vi "Pre Launch Init.vi"(11 "CS++DeviceGUIActor in":refnum<class "CS++DeviceGUIActor.lvclass">) -> (0 "error out":errorcluster, 3 "CS++DeviceGUIActor out":refnum<class "CS++DeviceGUIActor.lvclass">)   [LabVIEW 2013, in "CS++DeviceGUIActor.lvlib" / "CS++DeviceGUIActor.lvclass"]
doc: "(<B>Filename</B>: Actor Framework.lvlib:Actor.lvclass:Pre Launch Init.vi)\n\nDefines behavior that occurs after the Launch Actor method is invoked but before the actor's Actor Core method begins running.\n\nThe Pre Launch Init method is guaranteed to finish before the Launch Actor method returns to its caller and before the actor itself receives any messages. Any references that the Pre Launch Init method obtains are guaranteed to have the same lifetime as the actor itself. Any errors that the Pre Launch Init method returns will abort the launch.\n\nBy default, this method does nothing. A descendant class may override it to define behavior."
uses:
  CS++DeviceGUIActor.lvclass
  CS++GUIActor/CS++GUIActor.lvclass
  CS++BaseActor/CS++BaseActor.lvclass/CS++BaseActor.ctl
  Classes/CS++BaseClasses/Factory/CS++Factory.lvclass
  Classes/CS++ProcessVariables/PVConnection/PVConnection.lvclass
  Classes/CS++ProcessVariables/ProcessVariable/PV.lvclass/PV.ctl
  CS++DeviceGUIActor.lvclass/CS++DeviceGUIActor.ctl
  Classes/CS++ProcessVariables/ProcessVariable/Read Data.vi
  CS++BaseActor/Read CS++Factory.vi
  CS++GUIActor/Read Actor Name.vi
  Classes/CS++ProcessVariables/CS++ProcessVariables.lvlib
  Classes/CS++ProcessVariables/ProcessVariable/PV.lvclass
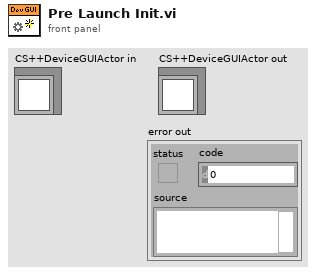
[diagram p1: front panel]
types:
  T1 = cluster{"Write Access":enum8{"Allowed", "Required", "None"}, "Read Access":enum8{"Allowed", "Required", "None"}}
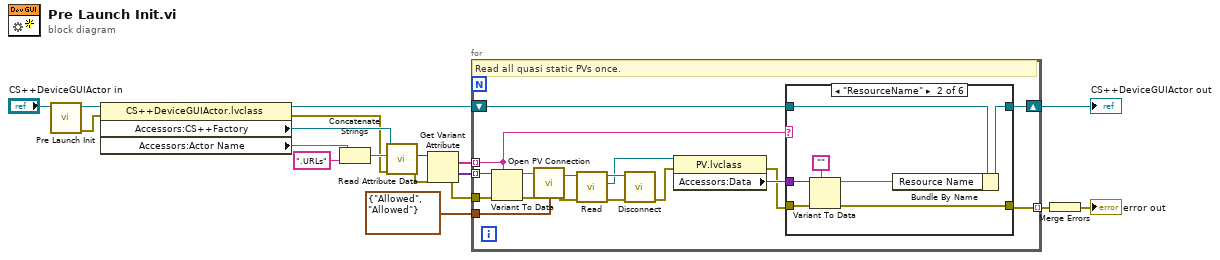
[diagram p0: block diagram]
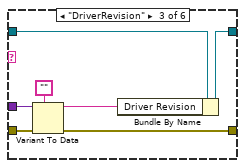
[diagram p3: hidden frame]
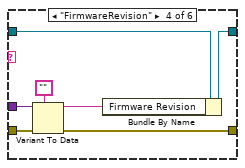
[diagram p4: hidden frame]
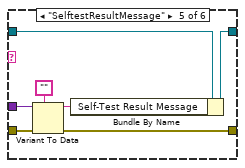
[diagram p5: hidden frame]
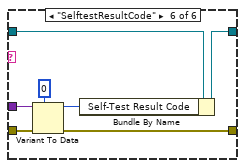
[diagram p6: hidden frame]
diagram:
  n1 = call-parent "Pre Launch Init.vi"("CS++BaseActor in"="CS++DeviceGUIActor in") -> ("error out"=w4:errorcluster, "CS++BaseActor out"=w5:refnum<class "CS++DeviceGUIActor.lvclass">)  [unwired: 9 in]
  n2 = property class="CS++DeviceGUIActor.lvclass"(reference=w5, error in=w4) -> (reference out=w7:refnum<class "CS++DeviceGUIActor.lvclass">, error out=w14:errorcluster, "Accessors:CS++Factory"=w15:refnum<class "CS++Factory.lvclass">, "Accessors:Actor Name"=w13:string)
  n3 = Concatenate Strings(w13, ".URLs" ("string")) -> (w16:string)
  n4 = call-dynamic "Read Attribute Data.vi"("error in (no error)"=w14, "Object Name"=w16, "CS++Factory in"=w15) -> ("error out"=w11:errorcluster, "Attribute Data"=w12:variant)  [unwired: 6 in, 1 out]
  n5 = Get Variant Attribute(Variant=w12, error in=w11) -> (names=w10:string[], values=w9:variant[], error out=w8:errorcluster)  [unwired: 2 in, 1 out]
  n6 = for {
    tunnel: w10 -> [w25] mode=indexing
    tunnel: w9 -> [w35] mode=indexing
    tunnel: w8 -> [w34]
    shift-right: [w32] -> w3
    shift-left: w7 -> [w33]
    tunnel: [w24] -> w6 mode=indexing
    tunnel: T1 {"Write Access"=enum."Allowed", "Read Access"=enum."Allowed"} ("Access (Read Required)") -> [w19]
    # "Read all quasi static PVs once."
    n7 = Variant To Data(error in=w34, type=w25, Variant=w35) -> (data=w23:string, error out=w22:errorcluster)
    n8 = call "Open PV Connection.vi"("PV URL"=w23, "Access (R/W allowed)"=w19, "Error In"=w22) -> ("PVConnection"=w21:refnum<class "PVConnection.lvclass">, "Error Out"=w20:errorcluster)
    n9 = call-dynamic "Read.vi"("error in (no error)"=w20, "PVConnection in"=w21) -> ("error out"=w30:errorcluster, "PV"=w29:refnum<class "PV.lvclass">, "PVConnection out"=w31:refnum<class "PVConnection.lvclass">)  [unwired: 6 in, 1 out]
    n10 = call-dynamic "Disconnect.vi"("error in (no error)"=w30, "PVConnection in"=w31) -> ("error out"=w28:errorcluster)  [unwired: 8 in, 1 out]
    n11 = property class="PV.lvclass"(reference=w29, error in=w28) -> (error out=w26:errorcluster, "Accessors:Data"=w27:variant)  [unwired: 1 out]
    n12 = case shown="\"ResourceName\"" w25 {
      tunnel: w33 -> [w37 w44 w51 w58 w65 w72]
      tunnel: [w37 w43 w50 w57 w64 w71] -> w32
      tunnel: w27 -> [_ w42 w49 w56 w63 w70]
      tunnel: w26 -> [w36 w40 w47 w54 w61 w68]
      tunnel: [w36 w38 w45 w52 w59 w66] -> w24
      frame Default {
      }
      frame "ResourceName" {
        n13 = Variant To Data(error in=w40, type="", Variant=w42) -> (data=w39:string, error out=w38:errorcluster)
        n14 = Bundle By Name(cluster=w44, "Resource Name"=w39) -> (w43:refnum<class "CS++DeviceGUIActor.lvclass">)
      }
      frame "DriverRevision" {
        n15 = Variant To Data(error in=w47, type="", Variant=w49) -> (data=w46:string, error out=w45:errorcluster)
        n16 = Bundle By Name(cluster=w51, "Driver Revision"=w46) -> (w50:refnum<class "CS++DeviceGUIActor.lvclass">)
      }
      frame "FirmwareRevision" {
        n17 = Variant To Data(error in=w54, type="", Variant=w56) -> (data=w53:string, error out=w52:errorcluster)
        n18 = Bundle By Name(cluster=w58, "Firmware Revision"=w53) -> (w57:refnum<class "CS++DeviceGUIActor.lvclass">)
      }
      frame "SelftestResultMessage" {
        n19 = Variant To Data(error in=w61, type="", Variant=w63) -> (data=w60:string, error out=w59:errorcluster)
        n20 = Bundle By Name(cluster=w65, "Self-Test Result Message"=w60) -> (w64:refnum<class "CS++DeviceGUIActor.lvclass">)
      }
      frame "SelftestResultCode" {
        n21 = Variant To Data(error in=w68, type=0, Variant=w70) -> (data=w67:i32, error out=w66:errorcluster)
        n22 = Bundle By Name(cluster=w72, "Self-Test Result Code"=w67) -> (w71:refnum<class "CS++DeviceGUIActor.lvclass">)
      }
    }
  }
  "CS++DeviceGUIActor out" <- w3
  n23 = Merge Errors(w6) -> (→"error out":errorcluster)
